vi "CSM - Register Broadcast.vi"(0 "CSM Name(Empty for Broadcast Event)":string, 5 "Source CSM Name (* as Default)":string="*", 7 "Trigger":string, 9 "API (If \"\", Same as Trigger)":string, 11 "Error In":errorcluster caption="error in (no error)", 12 "Priority(No Change)":T1) -> (4 "CSM Name (Dup)":string, 15 "error out":errorcluster)   [LabVIEW 2017, in "Communicable State Machine.lvlib"]
doc: "Registers to receive notifications of changes triggered by other CSM modules. If <b>API</b> is not wired or the input is empty, the trigger name will be used as the response message. The trigger name can be the broadcast name of the source module or the state name of the source module.\n\nIn Worker Mode and Chain of Responsibility Mode, the input node name is automatically parsed as the module name because CSM implements registrations on a per-module basis.\n\nReference Example: \"2. Caller is CSM Scenario\\CSM Example - Caller is a CSM.vi\".\n\n> [!NOTE] \n> <b>CSM Registration</b>\n>\n> Registration associates a broadcast with a bound interface (API). When the broadcast is triggered, the bound interface (API) is called. Registrations can also be cancelled. In CSM, there are two types of broadcasts:\n>\n> 1. <b>Broadcast:</b> Broadcast explicitly called by the module sending the broadcast message. Arguments need to be explicitly provided.\n> 2. <b>State:</b> Any state of a CSM module can also be registered to. The argument received by the triggered API is the Response of the CSM state.\n>\n> // Register `[Broadcast Message Name]@[SourceModule] >> [Bound API]@[TargetModule] -><register> // [Comments]`// Unregister `[Broadcast Message Name]@[SourceModule] >> [Bound API]@[TargetModule] -><unregister> // [Comments]`\n\n> - <b>Broadcast Message Name:</b> Defined by the source module. Refer to \"CSM Broadcast Format Parsing\" for details.\n> - <b>Source Module:</b> The broadcasting module. If subscribing to broadcasts from any module, the source module can be represented by `*`.\n> - <b>Bound API:</b> Defined by the target module. It is the external interface of the target module.\n> - <b>Target Module:</b> The module where the bound API resides. When indicating registration to the current module within a CSM module, it can be ignored. The preceding `@` separator is also omitted.\n> - `<register>` / `<unregister>`: Definition of the Register/Unregister operation type.\n> - <b>Comments:</b> Comment information, which will not be parsed.\n\n-- <b>Controls</b> --\n- <b>CSM Name</b>: CSM module name.\n- <b>Source CSM Name (* as Default)</b>: The CSM module generating the status. You can use \"*\" to represent all modules generating the same status.\n- <b>Trigger</b>: Trigger string.\n- <b>API (if \"\", same as Trigger)</b>: Upon registration, this message will be received if the trigger changes.\n\n-- <b>Indicators</b> --\n- <b>CSM Name (Dup)</b>: A copy of the input CSM module name."
uses:
  Communicable State Machine.lvlib
  CSM - Broadcast Message Type.ctl
  _Support/FGV-BroadcastRegistry/Operation-BroadcastRegistry.ctl
  _Support/GlobalEvent/GEvt-Generate with Rule Check.vi
  _Support/GlobalEvent/GEvt-Convert Filter Rules - v1.0.vi
  _Support/ChangeFlag/FlagInstance-GEvt Filter.vi
  _Support/ChangeFlag/ChangeFlag-Read.vi
  _Support/GlobalEvent/LogFilter/LogFilter - Check.vi
  _Support/GlobalEvent/LogFilter/SettingVIs/Set CSM StateType Filter.vi
  _Support/GlobalEvent/LogFilter/SettingVIs/Set Global StateType Filter.vi
  _Support/GlobalEvent/LogFilter/SettingVIs/Set CSM State Filter.vi
  _Support/GlobalEvent/LogFilter/SettingVIs/Set CSM LogType Filter.vi
  _Support/GlobalEvent/LogFilter/SettingVIs/Set Global State Filter.vi
  _Support/GlobalEvent/LogFilter/SettingVIs/Set Global LogType Filter.vi
  _Support/GlobalEvent/LogFilter/SettingVIs/Set Global CSM Filter.vi
  _Support/GlobalEvent/FGV-GEvt Filter Rules(lvlibp).vi
  _Support/ChangeFlag/ChangeFlagDB.vi
  _Support/GlobalEvent/LogFilter/LogFilter.lvclass
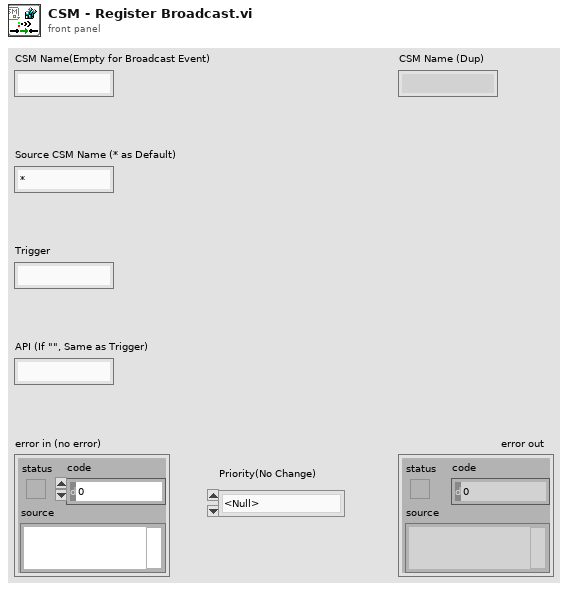
[diagram p1: front panel]
types:
  T1 = typedef "Communicable State Machine.lvlib/CSM - Broadcast Message Type.ctl" = enum16{"<Null>", "Status", "Interrupt"}
  T2 = typedef "Communicable State Machine.lvlib/Operation-BroadcastRegistry.ctl" = enum16{"Delete Source Module", "Delete Target Module", "Remove Module", "Register", "Unregister", "Check", "List Status", "List Entries", "List Status Of Source", "Drop", "Register As Status", "Register As Interrupt"}
  T3 = typedef "Communicable State Machine.lvlib/GEvt-Refs.ctl" = cluster{"Event":refnum<user-event>, "Queues":refnum<queue>[], "Valid":bool}
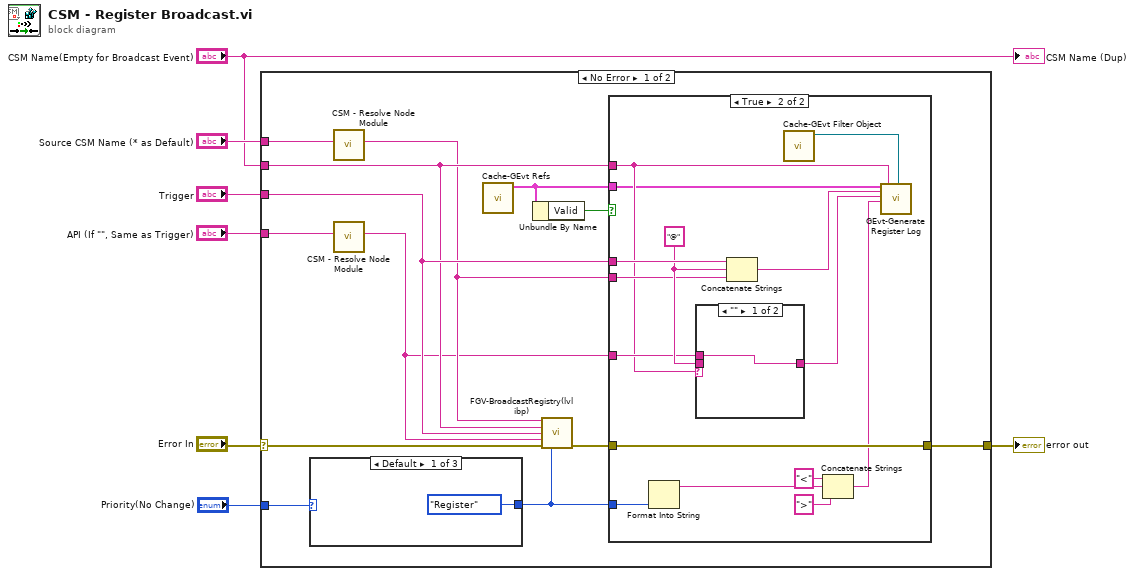
[diagram p0: block diagram]
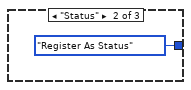
[diagram p2: hidden frame]
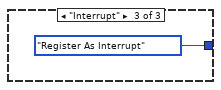
[diagram p3: hidden frame]
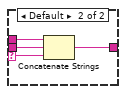
[diagram p5: hidden frame]
diagram:
  n1 = case shown="No Error" "Error In" {
    selector: "Error In" -> [w20 w45]
    tunnel: [w15 w45] -> w6
    tunnel: "API (If \"\", Same as Trigger)" -> [w18 _]
    tunnel: "Trigger" -> [w19 _]
    tunnel: "CSM Name(Empty for Broadcast Event)" -> [w16 _]
    tunnel: "Source CSM Name (* as Default)" -> [w17 _]
    tunnel: "Priority(No Change)" -> [w9 _]
    frame No Error {
      n2 = case shown="Default" w9 {
        tunnel: [Operation-BroadcastRegistry."Register" ("Operation") Operation-BroadcastRegistry."Register As Status" ("Operation") Operation-BroadcastRegistry."Register As Interrupt" ("Operation")] -> w8
        frame Default {
        }
        frame "Status" {
        }
        frame "Interrupt" {
        }
      }
      n3 = call "CSM - Resolve Node Module.vi"("Node Name"=w17) -> ("CSM Module Name"=w11:string)  [unwired: 10 in]
      n4 = call "CSM - Resolve Node Module.vi"("Node Name"=w18) -> ("CSM Module Name"=w10:string)  [unwired: 10 in]
      n5 = call "Cache-GEvt Refs.vi"() -> ("CSM Global Log Ref"=w13:T3)  [unwired: 10 in, 1 out]
      n6 = Unbundle By Name(w13) -> ("Valid"=w12:bool)
      n7 = call "FGV-BroadcastRegistry(lvlibp).vi"("Source"=w11, "Target"=w16, "Status"=w19, "API"=w10, "Error In"=w20, "Operation"=w8) -> ("error out"=w14:errorcluster)  [unwired: 7 in, 2 out]
      n8 = case shown="True" w12 {
        tunnel: w19 -> [_ w38]
        tunnel: w10 -> [_ w36]
        tunnel: w11 -> [_ w33]
        tunnel: w16 -> [_ w32]
        tunnel: w13 -> [_ w31]
        tunnel: [w24 w30] -> w15
        tunnel: w14 -> [w24 w30]
        tunnel: w8 -> [_ w29]
        frame False {
        }
        frame True {
          w37 = "@" ("string")
          n9 = Format Into String(w29) -> (resulting string=w28:string)  [unwired: 3 in, 1 out]
          n10 = case shown="\"\"" w32 {
            selector: w32 -> [_ w41]
            tunnel: w37 -> [_ w44]
            tunnel: w36 -> [w40 w43]
            tunnel: [w40 w42] -> w34
            frame "" {
            }
            frame Default {
              n11 = Concatenate Strings(w43, w44, w41) -> (w42:string)
            }
          }
          n12 = Concatenate Strings(w38, w37, w33) -> (w35:string)
          n13 = call "Cache-GEvt Filter Object.vi"() -> ("CSM:LogFilter.lvclass"=w39:refnum<class "LogFilter.lvclass">)  [unwired: 11 in]
          n14 = Concatenate Strings("<" ("string"), w28, ">" ("string")) -> (w27:string)
          n15 = call "GEvt-Generate Register Log.vi"("CSM Global Log Event"=w31, "Current State"=w35, "Arguments"=w34, "Source Module"=w27, "Name (\"\" to Use UUID)"=w32, "CSM:LogFilter.lvclass"=w39) -> ()  [unwired: 12 in, 2 out]
        }
      }
    }
    frame Error {
    }
  }
  "error out" <- w6
  "CSM Name (Dup)" <- "CSM Name(Empty for Broadcast Event)"
